vi "ImageFileAcquire.vi"(8 "error in":errorcluster, 10 "Index":i32, 11 "File Path":string) -> (0 "error out":errorcluster, 4 "return":i32)   [LabVIEW 2019]
uses:
  [Global] Image.vi
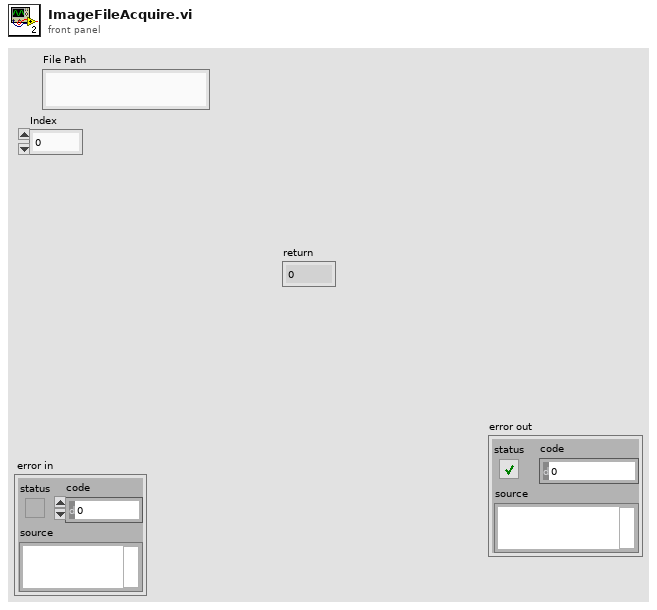
[diagram p1: front panel]
types:
  T1 = typedef "IMAQ Image.ctl" = refnum<image>
  T2 = typedef "Image Type" = u32
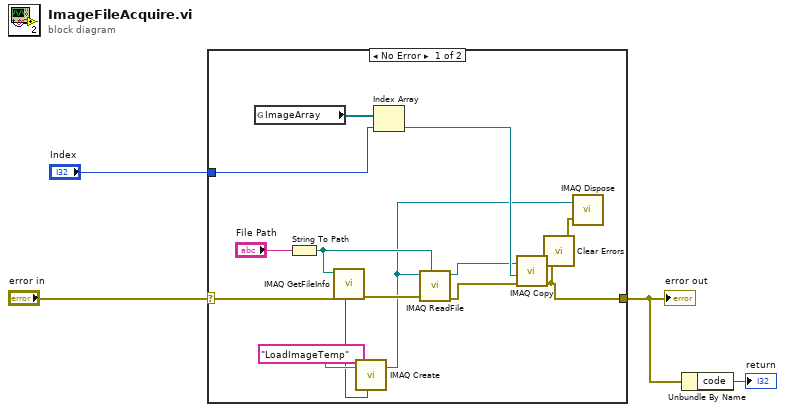
[diagram p0: block diagram]
diagram:
  n1 = case shown="No Error" "error in" {
    selector: "error in" -> [w15 w19]
    tunnel: [w7 w19] -> w1
    tunnel: "Index" -> [w16 _]
    frame No Error {
      n2 = global read "[Global] Image.vi" "ImageArray"() -> (w17:T1[])
      n3 = String To Path(string="File Path") -> (path=w13:path)
      n4 = call "IMAQ GetFileInfo"("error in (no error)"=w15, "File Path"=w13) -> ("error out"=w14:errorcluster, "Image Type"=w8:T2)  [unwired: 3 in, 5 out]
      n5 = call "IMAQ Create"("Image Name"="LoadImageTemp", "Image Type"=w8) -> ("New Image"=w5:T1)  [unwired: 3 in, 1 out]
      n6 = Index Array(array=w17, index=w16) -> (element=w12:T1)
      n7 = call "IMAQ ReadFile"("File Path"=w13, "error in (no error)"=w14, "Image"=w5) -> ("error out"=w11:errorcluster, "Image Out"=w10:T1)  [unwired: 4 in, 3 out]
      n8 = call "IMAQ Copy"("error in (no error)"=w11, "Image Dst"=w12, "Image Src"=w10) -> ("error out"=w7:errorcluster)  [unwired: 3 in, 1 out]
      n9 = call <vilib>:"Clear Errors.vi"("error in (no error)"=w7) -> ("error out"=w6:errorcluster)  [unwired: 5 in, 1 out]
      n10 = call "IMAQ Dispose"("Image"=w5, "error in (no error)"=w6) -> ()  [unwired: 4 in, 1 out]
    }
    frame Error {
    }
  }
  "error out" <- w1
  n11 = Unbundle By Name(w1) -> ("code"=→"return":i32)
